vi "Select.vi"(11 "Boolean":bool) -> (2 "0th row":dbl, 3 "1st row":dbl)   [LabVIEW 2014]
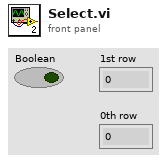
[diagram p1: front panel]
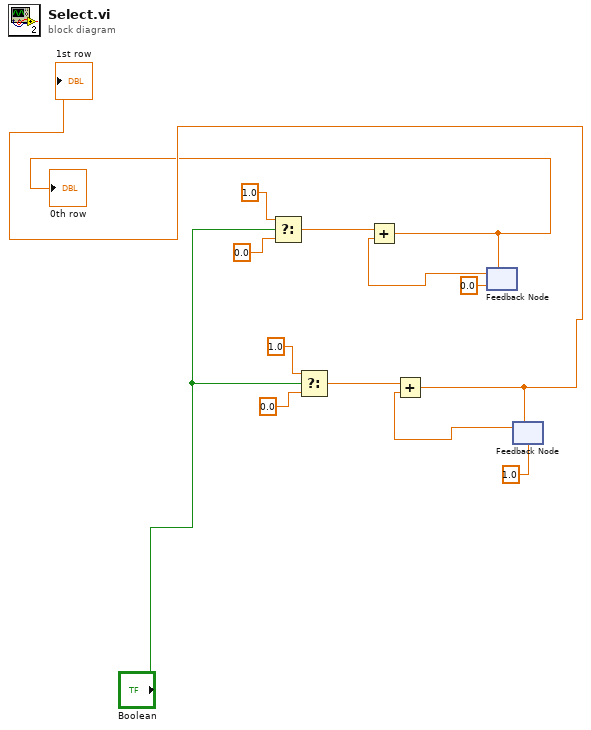
[diagram p0: block diagram]
diagram:
  n1 = Select(t=1.0, s="Boolean", f=0.0) -> (s? t:f=w3:dbl)
  n2 = Select(t=1.0, s="Boolean", f=0.0) -> (s? t:f=w9:dbl)
  n3 = feedback #1(0.0) -> (w4:dbl)
  n4 = Add(x=w3, y=w4) -> (x+y=w6:dbl)
  "0th row" <- w6
  n5 = feedback-in #1(w6) -> ()
  n6 = feedback #2(1.0) -> (w8:dbl)
  n7 = Add(x=w9, y=w8) -> (x+y=w13:dbl)
  "1st row" <- w13
  n8 = feedback-in #2(w13) -> ()
